vi "my_gpib_read.vi"(0 "address string":string, 5 "byte count":u32, 11 "error in":errorcluster) -> (4 "data":string, 15 "error out":errorcluster)   [LabVIEW 2019]
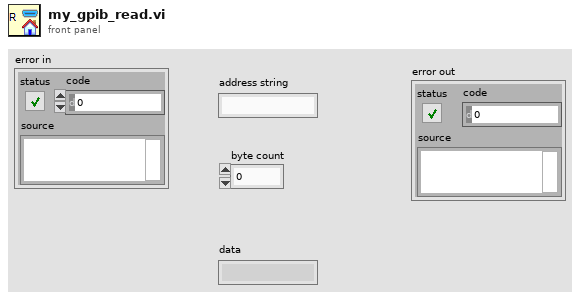
[diagram p1: front panel]
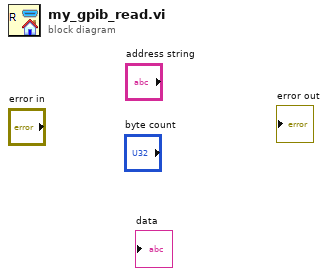
[diagram p0: block diagram]
diagram:
